vi "LCD Configure 4-bit.vi"(0 "Arduino Resource":T2, 7 "LCD Pin Config 4 Bit":T1={"RS"=12, "RW"=255, "Enable"=11, "D4"=5, "D5"=4, "D6"=3, "D7"=2, "LCD"=7}, 11 "error in":errorcluster) -> (4 "Arduino Resource":T2, 15 "error out":errorcluster)   [LabVIEW 2011, in "LabVIEW Interface for Arduino.lvlib"]
doc: "Configures the LCD according to the input pin configuration. A 4-bit setup configuration can be selected. If the RW pin is disconnected, or connected to ground, set the RW pin to 255."
uses:
  <vilib>/LabVIEW Interface for Arduino/LabVIEW Interface for Arduino.lvlib
  <vilib>/LabVIEW Interface for Arduino/Private/Type Defs/Arduino Resource.ctl
  <vilib>/LabVIEW Interface for Arduino/Private/Type Defs/Board Type.ctl
  <vilib>/LabVIEW Interface for Arduino/Private/Type Defs/LCD Pin Config 4 bit.ctl
  <vilib>/LabVIEW Interface for Arduino/Private/Type Defs/Command.ctl
  <vilib>/LabVIEW Interface for Arduino/Private/Type Defs/Pin Mode.ctl
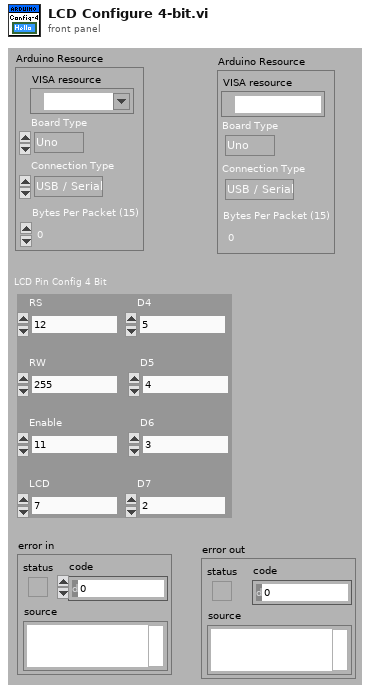
[diagram p1: front panel]
types:
  T1 = typedef "LabVIEW Interface for Arduino.lvlib/LCD Pin Config 4 bit.ctl" = cluster{"RS":u8, "RW":u8, "Enable":u8, "D4":u8, "D5":u8, "D6":u8, "D7":u8, "LCD":u8}
  T2 = typedef "LabVIEW Interface for Arduino.lvlib/Arduino Resource.ctl" = cluster{"VISA resource":refnum<visa-resource-name>, "Board Type":T3, "Connection Type":enum8{"USB / Serial"}, "Bytes Per Packet (15)":u8}
  T3 = typedef "LabVIEW Interface for Arduino.lvlib/Board Type.ctl" = enum16{"Uno", "Dimuelanove w/Atmega 328", "Mega 2560"}
  T4 = typedef "LabVIEW Interface for Arduino.lvlib/Pin Mode.ctl" = enum8{"Input", "Output"}
  T5 = typedef "LabVIEW Interface for Arduino.lvlib/Command.ctl" = enum8{"setArduinoMode", "flushSerial", "setPinMode", "digitalWritePin", "digitalWritePort", "tone", "digitalReadPin", "digitalReadPort", "analogReadPin", "analogReadPort", "pwmWritePin", "pwmWritePort", "sevenSegment_Configure", "sevenSegment_Write", "I2C Init", "I2C Write", "I2C Read", "SPI Init", "SPI Set Bit Order", "SPI Set Clock Divider", "SPI Set Data Mode", "SPI Send / Receive", "SPI Close", "Servo Set Num Servos", "Servo Config Servo", "Servo Write Angle", "Servo Read Angle", "Servo Write Pulse Width", "Servo Read Pulse Width", "Servo Detach", "LCD Init", "LCD Set Size", "LCD Set Cursor Mode", "LCD Clear", "LCD Set Cursor Position", "LCD Print", "LCD Display Power", "LCD Scroll Display", "LCD Autoscroll", "LCD Print Direction", "LCD Create Custom Char", "LCD Print Custom Char", "contAcqOn", "contAcqOff", "getFirmwareVersion", "FiniteSampleStart"}
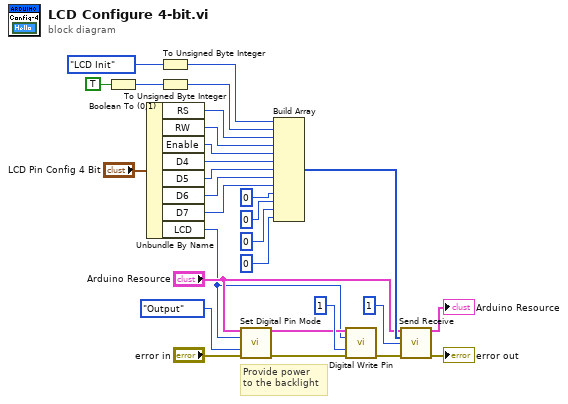
[diagram p0: block diagram]
diagram:
  # "Provide power\nto the backlight"
  n1 = Boolean To (0,1)(Boolean=TRUE) -> (0, 1=w17:i16)
  n2 = Unbundle By Name("LCD Pin Config 4 Bit") -> ("RS"=w18:u8, "RW"=w15:u8, "Enable"=w19:u8, "D4"=w20:u8, "D5"=w21:u8, "D6"=w22:u8, "D7"=w23:u8, "LCD"=w1:u8)
  n3 = To Unsigned Byte Integer(number=Command."LCD Init" ("Command")) -> (unsigned 8bit integer=w25:u8)
  n4 = To Unsigned Byte Integer(number=w17) -> (unsigned 8bit integer=w16:u8)
  n5 = call <vilib>:"Set Digital Pin Mode.vi"("Arduino Resource"="Arduino Resource", "Digital I/O Pin"=w1, "Pin Mode (Input)"=Pin_Mode."Output", "error in"="error in") -> ("Arduino Resource"=w7:T2, "error out"=w6:errorcluster)  [unwired: 10 in]
  n6 = Build Array(w25, w16, w18, w15, w19, w20, w21, w22, w23, u8 0 ("element"), u8 0 ("element"), u8 0 ("element"), u8 0 ("element")) -> (w26:u8[])
  n7 = call <vilib>:"Digital Write Pin.vi"("Arduino Resource"=w7, "Digital I/O Pin (0)"=w1, "Value (0)"=u8 1, "error in"=w6) -> ("error out"=w2:errorcluster)  [unwired: 10 in, 1 out]
  n8 = call <vilib>:"Send Receive.vi"("Arduino Resource"="Arduino Resource", "Data"=w26, "Bytes To Read (0)"=u8 1, "error in"=w2) -> ("Arduino Resource"=→"Arduino Resource":T2, "error out"=→"error out":errorcluster)  [unwired: 9 in, 1 out]
